vi "Get Topology.vi"(0 "SLSC Switch in":refnum<class "SLSC Switch.lvclass">, 5 "Topology Name In":string, 11 "error in (no error)":errorcluster) -> (4 "SLSC Switch out":refnum<class "SLSC Switch.lvclass">, 6 "Topology out":T1, 10 "Active Index":i32, 15 "error out":errorcluster)   [LabVIEW 2015, in "SLSC Switch.lvlib" / "SLSC Switch.lvclass"]
uses:
  SLSC Switch.lvclass
  <vilib>/SLSC/SLSC.lvlib
  Controls/JSON.InitialState.ctl
  Controls/JSON.ChannelList.ctl
  Controls/JSON.ConnectionList.ctl
  Controls/Topology.ctl
  <vilib>/SLSC/Unflatten Names (String).vi
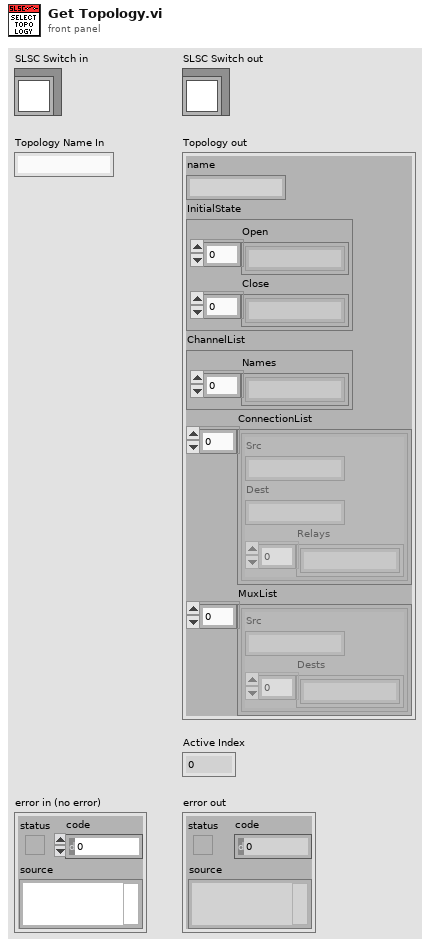
[diagram p1: front panel]
types:
  T1 = typedef "SLSC Switch.lvlib/SLSC Switch.lvclass/Topology.ctl" = cluster{"name":string, "InitialState":T2, "ChannelList":T3, "ConnectionList":T4[], "MuxList":cluster{"Src":string, "Dests":string[]}[]}
  T2 = typedef "SLSC Switch.lvlib/SLSC Switch.lvclass/JSON.InitialState.ctl" = cluster{"Open":string[], "Close":string[]}
  T3 = typedef "SLSC Switch.lvlib/SLSC Switch.lvclass/JSON.ChannelList.ctl" = cluster{"Names":string[]}
  T4 = typedef "SLSC Switch.lvlib/SLSC Switch.lvclass/JSON.ConnectionList.ctl" = cluster{"Src":string, "Dest":string, "Relays":string[]}
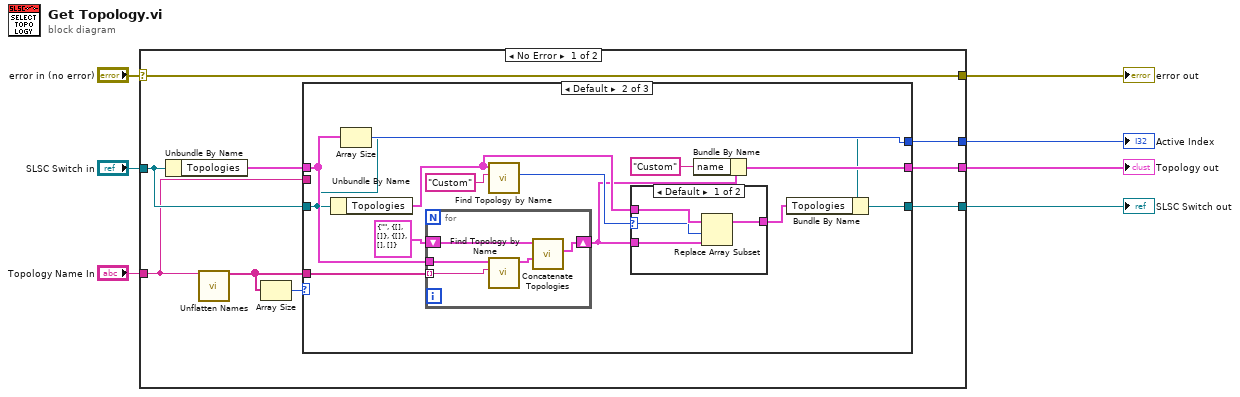
[diagram p0: block diagram]
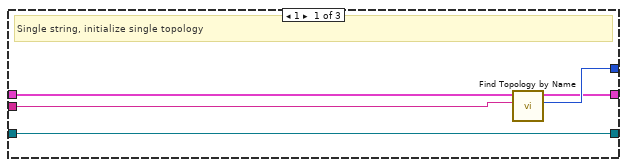
[diagram p2: hidden frame]
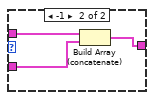
[diagram p3: hidden frame]
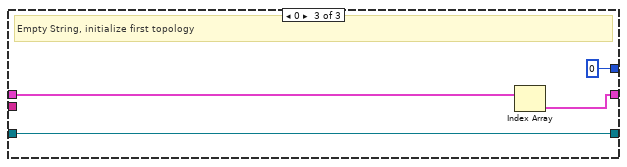
[diagram p4: hidden frame]
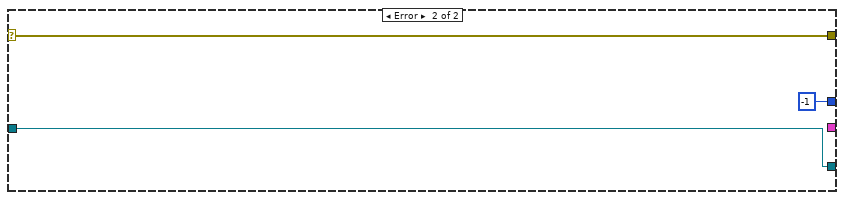
[diagram p5: hidden frame]
diagram:
  n1 = case shown="No Error" "error in (no error)" {
    selector: "error in (no error)" -> [w16 w53]
    tunnel: [w16 w53] -> w6
    tunnel: [w9 w52] -> w4
    tunnel: "SLSC Switch in" -> [w10 w52]
    tunnel: "Topology Name In" -> [w8 _]
    tunnel: [w14 _] -> w1
    tunnel: [w13 -1] -> w2
    frame No Error {
      n2 = Unbundle By Name(w10) -> ("Topologies"=w15:T1[])
      n3 = call-poly <vilib>:"Unflatten Names.vi"("names in"=w8) -> ("names out"=w11:string[])  [unwired: 13 in, 1 out]
      n4 = Array Size(array=w11) -> (size(s)=w12:i32)
      n5 = case shown="Default" w12 {
        tunnel: [w18 w28 w48] -> w14
        tunnel: [w19 w34 0] -> w13
        tunnel: w15 -> [w21 w31 w49]
        tunnel: w8 -> [w20 _ _]
        tunnel: w11 -> [_ w32 _]
        tunnel: w10 -> [w17 w27 w47]
        tunnel: [w17 w33 w47] -> w9
        frame 1 {
          # "Single string, initialize single topology"
          n6 = call "Find Topology by Name.vi"("Topology Name In"=w20, "Topologies"=w21) -> ("index"=w19:i32, "Topology"=w18:T1)  [unwired: 8 in]
        }
        frame Default {
          n7 = Unbundle By Name(w27) -> ("Topologies"=w25:T1[])
          n8 = Array Size(array=w31) -> (size(s)=w34:i32)
          n9 = for {
            tunnel: w32 -> [w46] mode=indexing
            tunnel: w31 -> [w45]
            shift-right: [w42] -> w24
            shift-left: T1 {"name"="", "InitialState"={"Open"=[], "Close"=[]}, "ChannelList"={"Names"=[]}, "ConnectionList"=[], "MuxList"=[]} ("Topology") -> [w44]
            n10 = call "Find Topology by Name.vi"("Topology Name In"=w46, "Topologies"=w45) -> ("Topology"=w43:T1)  [unwired: 8 in, 1 out]
            n11 = call "Concatenate Topologies.vi"("Topology B"=w43, "Topology A"=w44) -> ("Concatenated"=w42:T1)  [unwired: 9 in]
          }
          n12 = call "Find Topology by Name.vi"("Topology Name In"="Custom", "Topologies"=w25) -> ("index"=w26:i32)  [unwired: 8 in, 1 out]
          n13 = case shown="Default" w26 {
            selector: w26 -> [w37 _]
            tunnel: w25 -> [w38 w41]
            tunnel: w24 -> [w36 w40]
            tunnel: [w35 w39] -> w23
            frame Default {
              n14 = Replace Array Subset(array=w38, new element=w36, index=w37) -> (w35:T1[])
            }
            frame -1 {
              n15 = Build Array (concatenate)(w41, w40) -> (w39:T1[])
            }
          }
          n16 = Bundle By Name(cluster=w24, "name"="Custom") -> (w28:T1)
          n17 = Bundle By Name(cluster=w27, "Topologies"=w23) -> (w33:refnum<class "SLSC Switch.lvclass">)
        }
        frame 0 {
          # "Empty String, initialize first topology"
          n18 = Index Array(array=w49) -> (element=w48:T1)  [unwired: 1 in]
        }
      }
    }
    frame Error {
    }
  }
  "error out" <- w6
  "SLSC Switch out" <- w4
  "Active Index" <- w2
  "Topology out" <- w1
